vi "Configure Measurement.vi"(8 "error in (no error)":errorcluster, 10 "Function (0: Cp-D)":T1, 11 "LCR Meter in":refnum<class "LCR Meter.lvclass">) -> (0 "error out":errorcluster, 3 "LCR Meter out":refnum<class "LCR Meter.lvclass">)   [LabVIEW 2020, in "LCR Meter.lvclass"]
uses:
  LCR Meter.lvclass
  Controls/Function.ctl
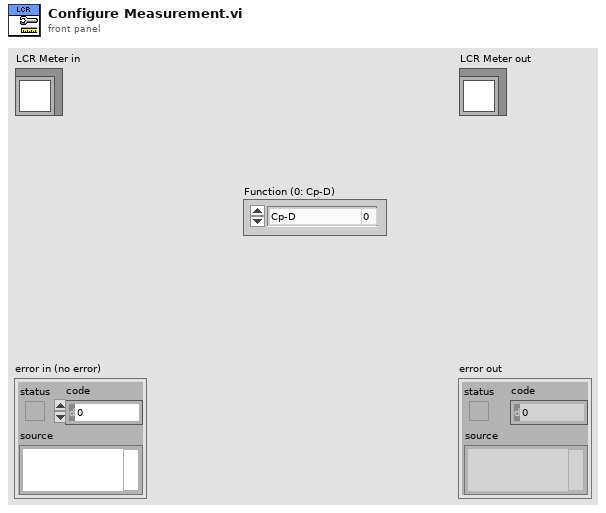
[diagram p1: front panel]
types:
  T1 = typedef "LCR Meter.lvclass/Function.ctl" = enum16{"Cp-D", "Cp-Q", "Cp-G", "Cp-Rp", "Cs-D", "Cs-Q", "Cs-Rs", "Lp-D", "Lp-Q", "Lp-G", "Lp-Rp", "Lp-Rdc", "Ls-D", "Ls-Q", "Ls-Rs", "Ls-Rdc", "R-X", "Z-thd", "Z-thr", "G-B", "Y-thd", "Y-thr", "Vdc-Idc"}
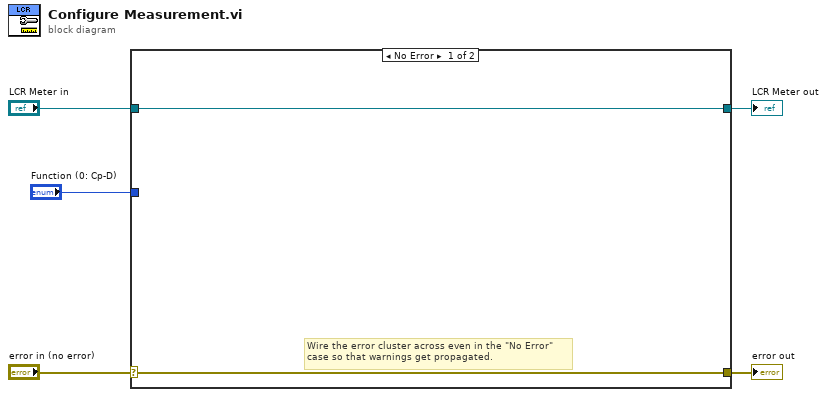
[diagram p0: block diagram]
diagram:
  n1 = case shown="No Error" "error in (no error)" {
    selector: "error in (no error)" -> [w6 w9]
    tunnel: [w6 w9] -> w4
    tunnel: [w7 w8] -> w2
    tunnel: "LCR Meter in" -> [w7 w8]
    tunnel: "Function (0: Cp-D)" -> [_ _]
    frame No Error {
      # "Wire the error cluster across even in the \"No Error\"\ncase so that warnings get propagated."
    }
    frame Error {
    }
  }
  "error out" <- w4
  "LCR Meter out" <- w2
